vi "Update State.vi"(11 "Great Wall in":refnum<class "Great Wall.lvclass">) -> (3 "Great Wall out":refnum<class "Great Wall.lvclass">)   [LabVIEW 2020, in "Great Wall.lvclass"]
uses:
  Great Wall.lvclass
  Great Wall.lvclass/Great Wall.ctl
  SubVIs/Read-Only Globals.vi
  SubVIs/Globals (private).vi
  Square/Square.lvclass
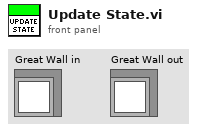
[diagram p1: front panel]
types:
  T1 = typedef "Great Wall.lvclass/Private Data.ctl" = cluster{"wall 1":T2, "wall 2":T2, "start row":i32, "start col":i32, "state update round":i32}
  T2 = typedef "Great Wall.lvclass/Wall State.ctl" = cluster{"state":T3, "direction":T4, "index":i32}
  T3 = typedef "Great Wall.lvclass/Wall State Enum.ctl" = enum16{"Under Construction", "Hold", "Advance 1", "Advance 2", "Retreat"}
  T4 = typedef "SB Type Defs.lvlib/Direction Enum.ctl" = enum16{"NW", "N", "NE", "E", "SE", "S", "SW", "W"}
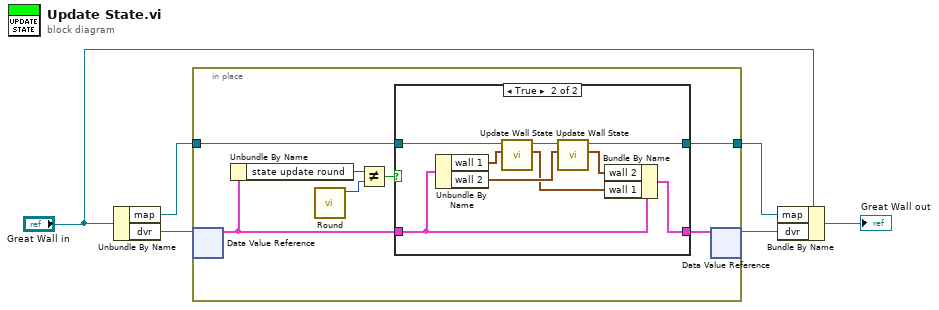
[diagram p0: block diagram]
diagram:
  n1 = Unbundle By Name("Great Wall in") -> ("map"=w2:refnum<data-value>, "dvr"=w6:refnum<data-value>)
  n2 = in-place {
    in-place-border: w2 -> [w8]
    in-place-border: [w7] -> w1
    n3 = in-place-dvr #1(w6) -> (w10:T1)  [unwired: 1 out]
    n4 = Unbundle By Name(w10) -> ("state update round"=w13:i32)
    n5 = call "Round.vi"() -> ("Round"=w12:i32)  [unwired: 11 in]
    n6 = Not Equal?(x=w13, y=w12) -> (x != y?=w11:bool)
    n7 = case shown="True" w11 {
      tunnel: w10 -> [w15 w20]
      tunnel: [w15 w16] -> w9
      tunnel: w8 -> [w14 w24]
      tunnel: [w14 w17] -> w7
      frame False {
      }
      frame True {
        n8 = Unbundle By Name(w20) -> ("wall 1"=w23:T2, "wall 2"=w21:T2)
        n9 = call "Update Wall State.vi"("wall state in"=w23, "map in"=w24) -> ("wall state out"=w18:T2, "map out"=w22:refnum<data-value>)  [unwired: 8 in]
        n10 = call "Update Wall State.vi"("wall state in"=w21, "map in"=w22) -> ("wall state out"=w19:T2, "map out"=w17:refnum<data-value>)  [unwired: 8 in]
        n11 = Bundle By Name(cluster=w20, "wall 2"=w19, "wall 1"=w18) -> (w16:T1)
      }
    }
    n12 = in-place-dvr #1(w9) -> (w3:refnum<data-value>)  [unwired: 1 out]
  }
  n13 = Bundle By Name(cluster="Great Wall in", "map"=w1, "dvr"=w3) -> (→"Great Wall out":refnum<class "Great Wall.lvclass">)
